vi "Transceiver.Get Class.vi"(8 "error in (no error)":errorcluster, 11 "Transceiver in":refnum<class "Transceiver.lvclass">) -> (0 "error out":errorcluster, 2 "class":string, 3 "Transceiver out":refnum<class "Transceiver.lvclass">)   [LabVIEW 2017, in "DSF Core.lvlib" / "Transceiver.lvclass"]
uses:
  Transceiver.lvclass
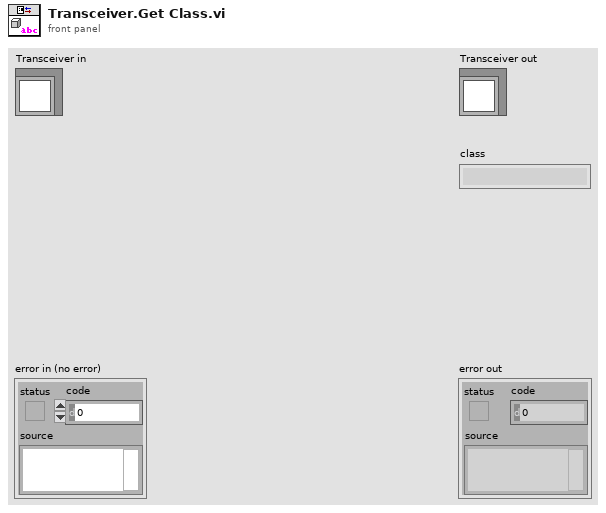
[diagram p1: front panel]
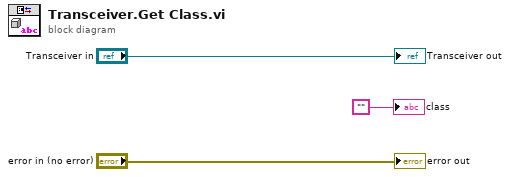
[diagram p0: block diagram]
diagram:
  "error out" <- "error in (no error)"
  "Transceiver out" <- "Transceiver in"
  "class" <- ""
